vi "UDP_send_conditional_v04.vi"() -> ()   [LabVIEW 2025]
uses:
  <vilib>/Utility/file.llb/Write Delimited Spreadsheet (DBL).vi
panel:
  in  "EEG_Channels_N":i32
  in  "EMG_Channels_N":i32
  in  "append to file? (new file:F) 2":bool
  in  "append to file? (new file:F)":bool
  in  "stop":bool
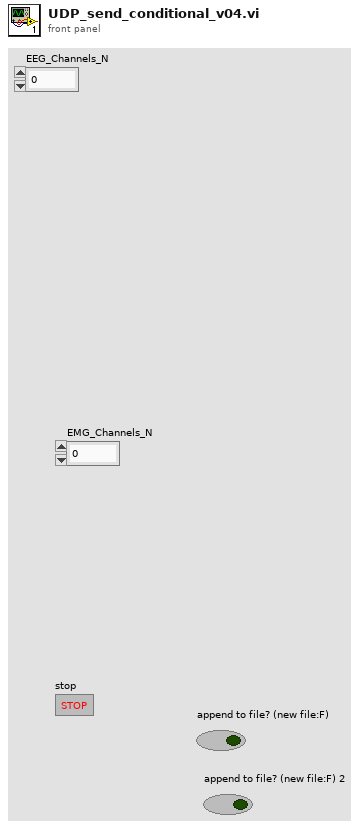
[diagram p1: front panel]
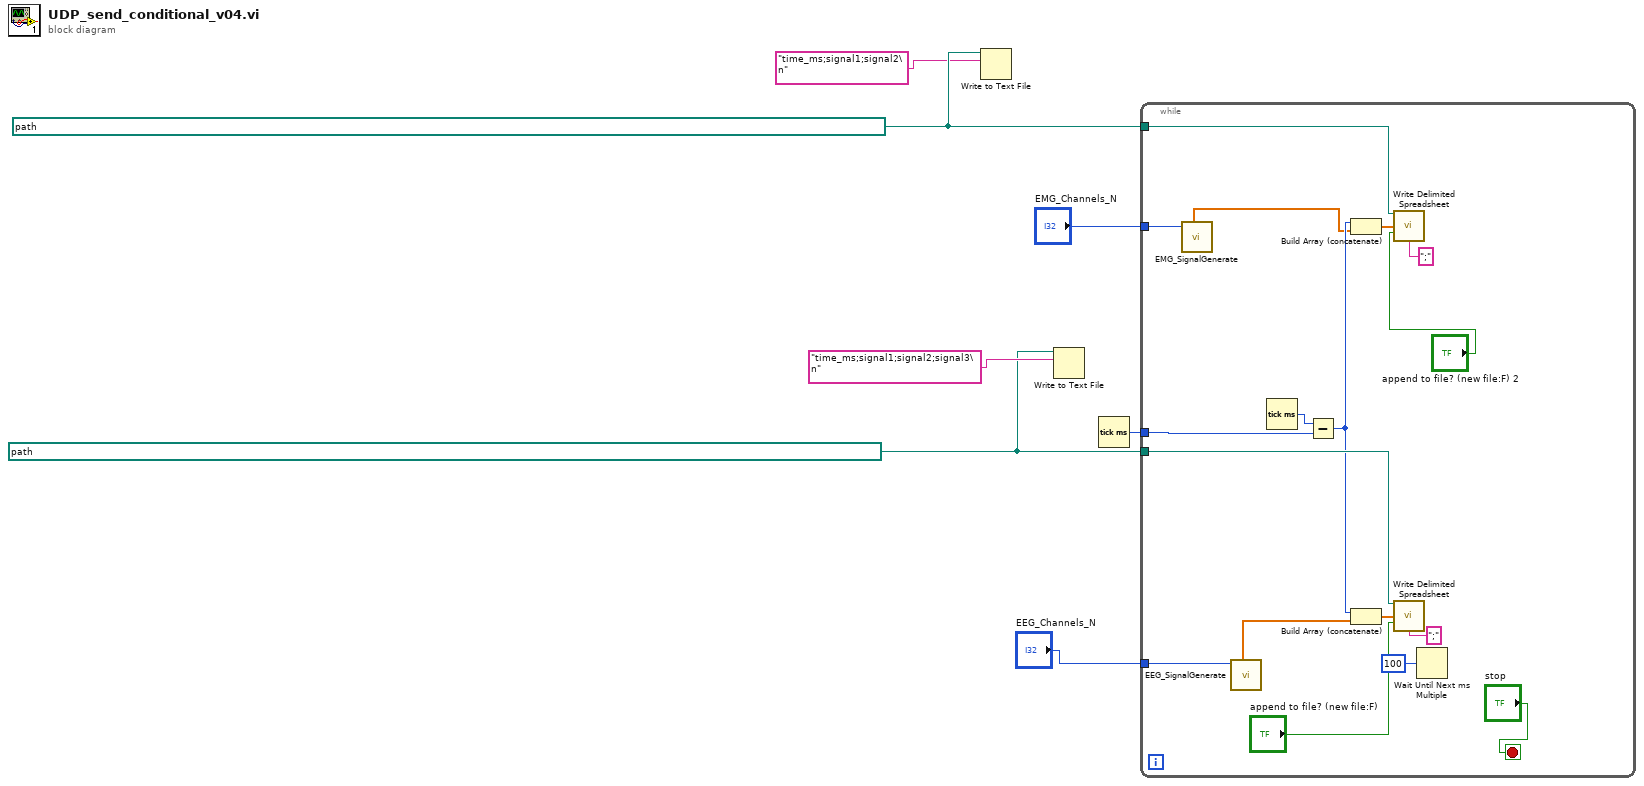
[diagram p0: block diagram]
diagram:
  w6 = path "G:/Meu Drive/Documentos/Academic/UFU/Estágios/Internship Italy/Classes/Graphical Programming LabVIEW (Prof. Calogero Oddo)/Final Project/test_signal2.csv" ("file path (dialog if empty)")
  w3 = path "G:/Meu Drive/Documentos/Academic/UFU/Estágios/Internship Italy/Classes/Graphical Programming LabVIEW (Prof. Calogero Oddo)/Final Project/test_signal1.csv" ("file path (dialog if empty)")
  n1 = Write to Text File(file (use dialog)=w6, text="time_ms;signal1;signal2\n") -> ()  [unwired: 2 in, 3 out]
  n2 = Write to Text File(file (use dialog)=w3, text="time_ms;signal1;signal2;signal3\n") -> ()  [unwired: 2 in, 3 out]
  n3 = Tick Count (ms)() -> (millisecond timer value=w7:u32)
  n4 = while {
    tunnel: w3 -> [w23]
    tunnel: w7 -> [w20]
    tunnel: w6 -> [w17]
    tunnel: "EMG_Channels_N" -> [w10]
    tunnel: "EEG_Channels_N" -> [w8]
    stop <- "stop" stop-if-true
    n5 = call "EMG_SignalGenerate.vi"("EMG_Channels_N"=w10) -> ("Array"=w11:dbl[])  [unwired: 10 in]
    n6 = call "EEG_SignalGenerate.vi"("EEG_Channels_N"=w8) -> ("Array"=w9:dbl[])  [unwired: 10 in]
    n7 = Tick Count (ms)() -> (millisecond timer value=w19:u32)
    n8 = Subtract(x=w19, y=w20) -> (x-y=w15:u32)
    n9 = Build Array (concatenate)(w15, w11) -> (w14:dbl[])
    n10 = Build Array (concatenate)(w15, w9) -> (w21:dbl[])
    n11 = call-poly <vilib>:"Write Delimited Spreadsheet.vi"("file path (dialog if empty)"=w17, "1D data"=w14, "append to file? (new file:F)"="append to file? (new file:F) 2", "delimiter (\\t)"=";" ("delimiter (\\t)")) -> ()  [unwired: 10 in, 2 out]
    n12 = call-poly <vilib>:"Write Delimited Spreadsheet.vi"("file path (dialog if empty)"=w23, "1D data"=w21, "append to file? (new file:F)"="append to file? (new file:F)", "delimiter (\\t)"=";" ("delimiter (\\t)")) -> ()  [unwired: 10 in, 2 out]
    n13 = Wait Until Next ms Multiple(millisecond multiple=u32 100) -> ()  [unwired: 1 out]
  }
